vi "DMM Measurement.vi"() -> ()   [LabVIEW 2021]
doc: "This example acquires a single measurement from a National Instruments DMM. Select the measurement function and range. Specify the resolution in digits of precision. The measured value will be displayed in the Measurement indicator. The Boolean indicator will indicate if the measured value is out of range."
uses:
  <instrlib>/niDMM/nidmm.llb/niDMM Configure Measurement Digits.vi
  <instrlib>/niDMM/nidmm.llb/niDMM Function.ctl
  <instrlib>/niDMM/nidmm.llb/niDMM Resolution in Digits.ctl
panel:
  out "Load Voltage":dbl caption="SMU Measurement" format="%.6p"
  in  "SMU Range":dbl=10.0 format="%.2f"
  in  "Load DMM":refnum<k15>="Dev1"
  out "Load DMM Out of Range":bool caption="SMU Signal Out of Range"
  in  "Load DMM Measurement":T1 caption="SMU DMM Measurement"
  out "Load DMM Voltage":dbl caption="SMU Absolute Resolution" format="%#_3p"
  in  "Load DMM Resolution":T2=5.5 caption="SMU Resolution in Digits" items=["3 1/2"=3.5, "4 1/2"=4.5, "5 1/2"=5.5, "6 1/2"=6.5, "7 1/2"=7.5]
  out "error out":errorcluster
  in  "error in":errorcluster caption="error in (no error)"
  in  "SMU Resolution in Digits":T2=5.5 items=["3 1/2"=3.5, "4 1/2"=4.5, "5 1/2"=5.5, "6 1/2"=6.5, "7 1/2"=7.5]
  out "SMU DMM Resolution":dbl caption="SMU Absolute Resolution" format="%#_3p"
  in  "SMU DMM Measurement":T1
  out "SMU DMM Out of Range":bool caption="SMU Signal Out of Range"
  in  "SMU Range":dbl=10.0 format="%.2f"
  in  "SMU DMM":refnum<k15>="Dev1"
  out "SMU Measurement":dbl format="%.6p"
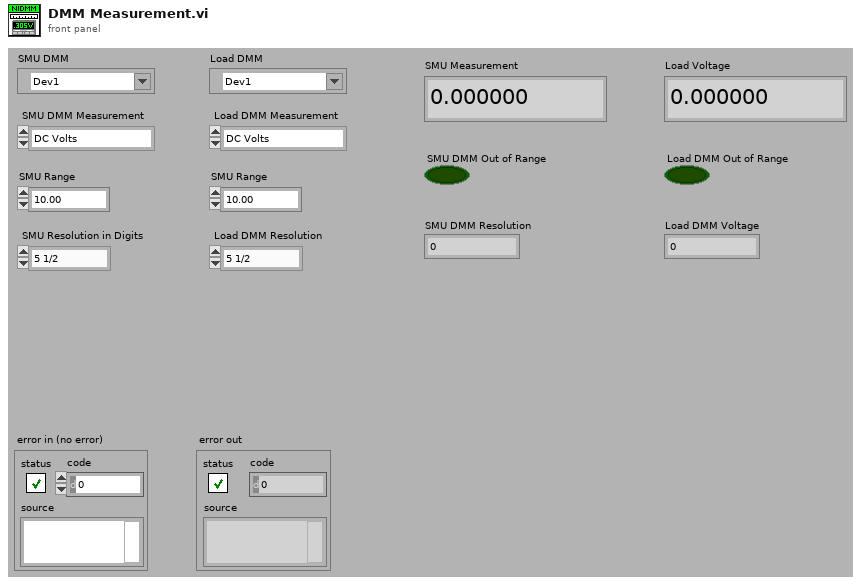
[diagram p1: front panel]
types:
  T1 = typedef "niDMM Function.ctl" = enum16{"DC Volts", "AC Volts", "DC Current", "AC Current", "2-wire Resistance", "4-wire Resistance", "Diode", "Frequency", "Period", "AC Volts DC Coupled", "Capacitance", "Inductance", "Temperature"}
  T2 = typedef "niDMM Resolution in Digits.ctl" = dbl
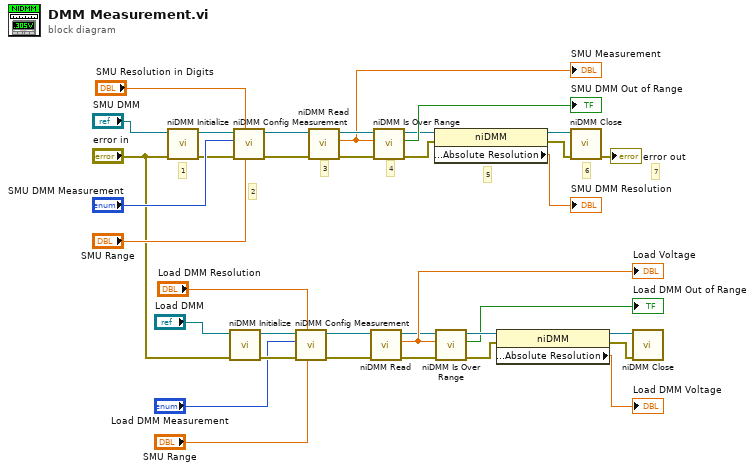
[diagram p0: block diagram]
diagram:
  # "2"
  # "1"
  # "7"
  # "6"
  # "5"
  # "4"
  # "3"
  n1 = call <instrlib>:"niDMM Initialize.vi"("error in (no error)"="error in", "Instrument Descriptor"="SMU DMM") -> ("error out"=w28:errorcluster, "instrument handle out"=w27:refnum<k15>)  [unwired: 8 in]
  n2 = call <instrlib>:"niDMM Initialize.vi"("error in (no error)"="error in", "Instrument Descriptor"="Load DMM") -> ("error out"=w12:errorcluster, "instrument handle out"=w13:refnum<k15>)  [unwired: 8 in]
  n3 = call-poly <instrlib>:"niDMM Config Measurement.vi"("Range"="SMU Range", "Resolution in Digits"="SMU Resolution in Digits", "error in (no error)"=w28, "Function"="SMU DMM Measurement", "instrument handle"=w27) -> ("error out"=w35:errorcluster, "instrument handle out"=w34:refnum<k15>)  [unwired: 5 in]
  n4 = call-poly <instrlib>:"niDMM Config Measurement.vi"("Range"="SMU Range", "Resolution in Digits"="Load DMM Resolution", "error in (no error)"=w12, "Function"="Load DMM Measurement", "instrument handle"=w13) -> ("error out"=w5:errorcluster, "instrument handle out"=w6:refnum<k15>)  [unwired: 5 in]
  n5 = call <instrlib>:"niDMM Read.vi"("error in (no error)"=w35, "instrument handle"=w34) -> ("error out"=w32:errorcluster, "Measurement"=w30:dbl, "instrument handle out"=w33:refnum<k15>)  [unwired: 7 in]
  "SMU Measurement" <- w30
  n6 = call <instrlib>:"niDMM Read.vi"("error in (no error)"=w5, "instrument handle"=w6) -> ("error out"=w8:errorcluster, "Measurement"=w10:dbl, "instrument handle out"=w7:refnum<k15>)  [unwired: 7 in]
  "Load Voltage" <- w10
  n7 = call <instrlib>:"niDMM Is Over Range.vi"("error in (no error)"=w32, "Measurement"=w30, "instrument handle"=w33) -> ("error out"=w24:errorcluster, "Over Range?"=→"SMU DMM Out of Range":bool, "instrument handle out"=w26:refnum<k15>)  [unwired: 6 in]
  n8 = property class="niDMM"(reference=w26, error in=w24) -> (reference out=w25:refnum<k15>, error out=w23:errorcluster, "Configuration:Absolute Resolution"=→"SMU DMM Resolution":dbl)
  n9 = call <instrlib>:"niDMM Is Over Range.vi"("error in (no error)"=w8, "Measurement"=w10, "instrument handle"=w7) -> ("error out"=w16:errorcluster, "Over Range?"=→"Load DMM Out of Range":bool, "instrument handle out"=w14:refnum<k15>)  [unwired: 6 in]
  n10 = property class="niDMM"(reference=w14, error in=w16) -> (reference out=w15:refnum<k15>, error out=w17:errorcluster, "Configuration:Absolute Resolution"=→"Load DMM Voltage":dbl)
  n11 = call <instrlib>:"niDMM Close.vi"("error in (no error)"=w23, "instrument handle"=w25) -> ("error out"=→"error out":errorcluster)  [unwired: 9 in]
  n12 = call <instrlib>:"niDMM Close.vi"("error in (no error)"=w17, "instrument handle"=w15) -> ()  [unwired: 9 in, 1 out]
